vi "Write RunTime.vi"(7 "Send any changes now? (F)":bool, 8 "error in (no error)":errorcluster, 9 "Start time":bool, 10 "Run Time":T1, 11 "Fiber Auto Collimation state data in":refnum<class "Fiber Auto Collimation state data.lvclass">) -> (0 "error out":errorcluster, 3 "Fiber Auto Collimation state data out":refnum<class "Fiber Auto Collimation state data.lvclass">)   [LabVIEW 2018, in "Fiber Auto Collimation state data.lvclass"]
doc: "Serial number of the Device Under Test on the station at the moment."
uses:
  Fiber Auto Collimation state data.lvclass
  Run Time.ctl
  Fiber Auto Collimation state data.lvclass/Fiber Auto Collimation state data.ctl
  Tracked state data.ctl
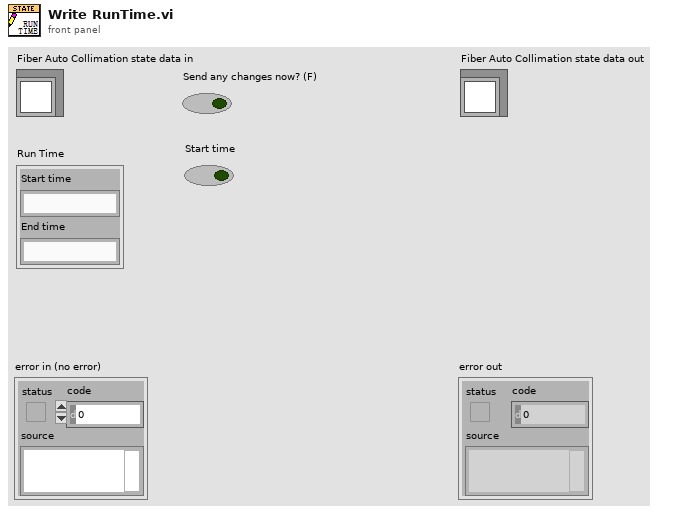
[diagram p1: front panel]
types:
  T1 = typedef "Fiber Auto Collimation state data.lvclass/Run Time.ctl" = cluster{"Start time":string, "End time":string}
  T2 = typedef "Fiber Auto Collimation state data.lvclass/Tracked state data.ctl" = enum16{"No update", "Permission level", "Username", "Test running", "DUT Serial", "Test status", "MOM Lot", "Loaded test recipe", "Model case running", "Station status", "BV data", "Defect Identify data", "Axis Position data", "Fiber Ass PN", "Operator", "RunTime", "VBAI", "Steps Cycle Time"}
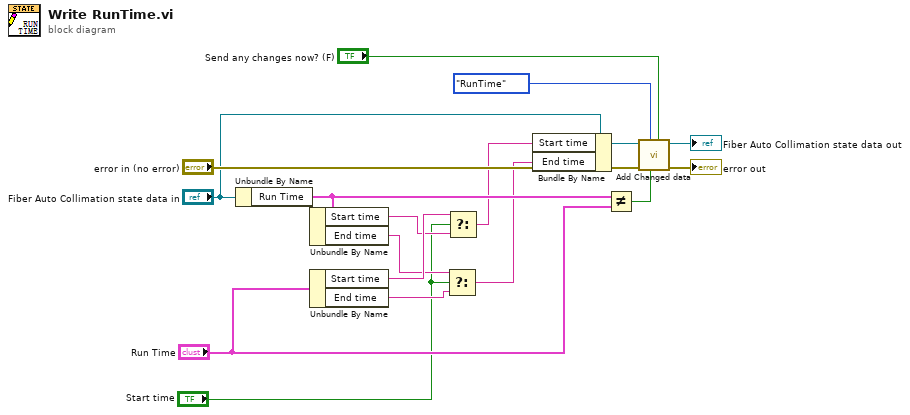
[diagram p0: block diagram]
diagram:
  n1 = Unbundle By Name("Fiber Auto Collimation state data in") -> ("Run Time"=w8:cluster{"Start time":string, "End time":string})
  n2 = Unbundle By Name(w8) -> ("Start time"=w6:string, "End time"=w4:string)
  n3 = Unbundle By Name("Run Time") -> ("Start time"=w7:string, "End time"=w3:string)
  n4 = Select(t=w4, s="Start time", f=w3) -> (s? t:f=w1:string)
  n5 = Select(t=w7, s="Start time", f=w6) -> (s? t:f=w5:string)
  n6 = Bundle By Name(cluster="Fiber Auto Collimation state data in", "Start time"=w5, "End time"=w1) -> (w14:refnum<class "Fiber Auto Collimation state data.lvclass">)
  n7 = Not Equal?(x=w8, y="Run Time") -> (x != y?=w11:bool)
  n8 = call "Add Changed data.vi"("Send any changes now? (F)"="Send any changes now? (F)", "Data changed?"=w11, "Data type"=Tracked_state_data."RunTime", "error in (no error)"="error in (no error)", "Fiber Auto Collimation state data in"=w14) -> ("error out"=→"error out":errorcluster, "Fiber Auto Collimation state data out"=→"Fiber Auto Collimation state data out":refnum<class "Fiber Auto Collimation state data.lvclass">)  [unwired: 5 in]
